vi "sub_ini-heading_from_nmea-log.vi"(11 "Log_nmea":string) -> (2 "init heading":dbl, 3 "init tm":cluster{"Lat":dbl, "Long":dbl})   [LabVIEW 2019]
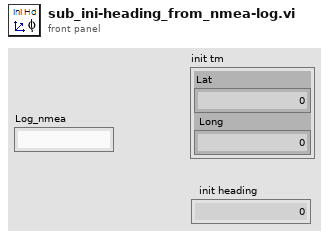
[diagram p1: front panel]
types:
  T1 = enum16{"GxDTM", "GxGBS", "GxGGA", "GxGLL", "GxGNS", "GxGRS", "GxGSA", "GxGST", "GxGSV", "GxRLM", "GxRMC", "GxTHS", "GxTXT", "GxVLW", "GxVTG", "GxZDA"}
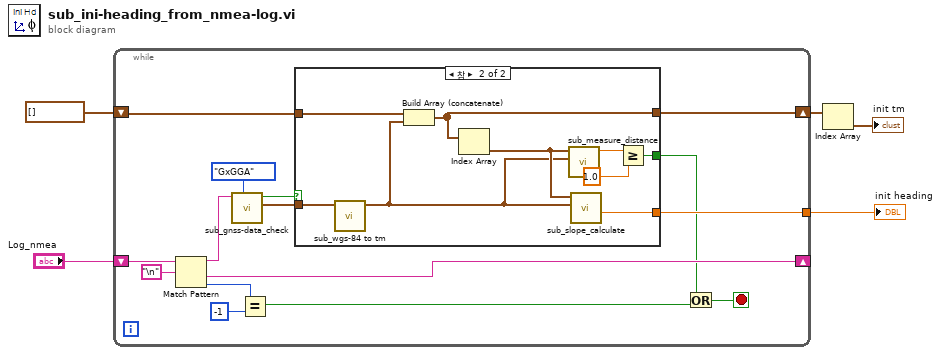
[diagram p0: block diagram]
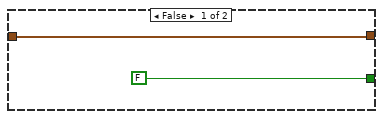
[diagram p2: hidden frame]
diagram:
  n1 = while {
    shift-right: [w17] -> _
    shift-left: "Log_nmea" -> [w18]
    shift-right: [w14] -> w2
    shift-left: cluster{"Lat":dbl, "Long":dbl}[] [] -> [w15]
    tunnel: [w13] -> w5
    stop <- w8 stop-if-true
    n2 = Match Pattern(string=w18, regular expression="\n") -> (before substring=w16:string, after substring=w17:string, offset past match=w11:i32)  [unwired: 1 in, 1 out]
    n3 = call "sub_gnss-data_check.vi"("sel"=T1."GxGGA", "gnss str"=w16) -> ("LatLong"=w7:cluster{dbl, dbl}, "val"=w6:bool)  [unwired: 7 in, 1 out]
    n4 = Equal?(x=w11, y=-1) -> (x = y?=w9:bool)
    n5 = case shown="참" w6 {
      tunnel: w7 -> [_ w24]
      tunnel: w15 -> [w22 w31]
      tunnel: [w22 w30] -> w14
      tunnel: [FALSE w27] -> w12
      tunnel: [_ w25] -> w13
      frame False {
      }
      frame True {
        n6 = call "sub_wgs-84 to tm.vi"("in_lon-lat"=w24) -> ("TM"=w23:cluster{"Y(E)":dbl, "X(N)":dbl})  [unwired: 10 in]
        n7 = Build Array (concatenate)(w31, w23) -> (w30:cluster{"Y(E)":dbl, "X(N)":dbl}[])
        n8 = Index Array(array=w30) -> (element=w26:cluster{"Y(E)":dbl, "X(N)":dbl})  [unwired: 1 in]
        n9 = call "sub_measure_distance.vi"("pt 2"=w23, "pt 1"=w26) -> ("distance"=w29:dbl)  [unwired: 9 in]
        n10 = call "sub_slope_calculate.vi"("point n+1"=w23, "point n"=w26) -> ("deg_gps-base"=w25:dbl)  [unwired: 7 in, 2 out]
        n11 = Greater Or Equal?(x=w29, y=1.0) -> (x >= y?=w27:bool)
      }
    }
    n12 = Or(x=w12, y=w9) -> (x .or. y?=w8:bool)
  }
  "init heading" <- w5
  n13 = Index Array(array=w2) -> (element=→"init tm":cluster{"Y(E)":dbl, "X(N)":dbl})  [unwired: 1 in]
